vi "Without Data.vi"(8 "Error In":errorcluster, 11 "Communication In":refnum<class "Communication.lvclass">) -> (0 "Error Out":errorcluster, 3 "Communication Out":refnum<class "Communication.lvclass">)   [LabVIEW 2022 SP3, in "Communication.lvclass"]
doc: "This VI is an overriding method which notify the receiver without any data."
uses:
  Communication.lvclass
  Downloads/Sample PC Template/Sample PC Template/Typedefs/Data.ctl
  Downloads/Sample PC Template/Sample PC Template/Sample PC Template.lvlib
  Controls/User Event Operation.ctl
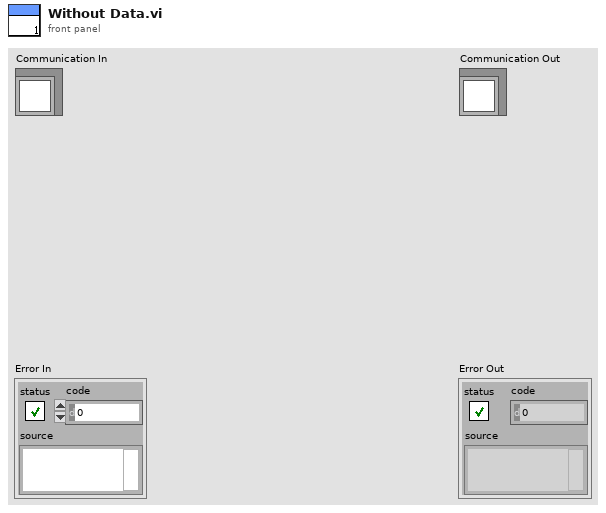
[diagram p1: front panel]
types:
  T1 = typedef "User Event Operation.ctl" = enum16{"Obtain", "Generate", "Release"}
  T2 = typedef "Sample PC Template.lvlib/Data.ctl" = cluster{"State":string, "Data":variant}
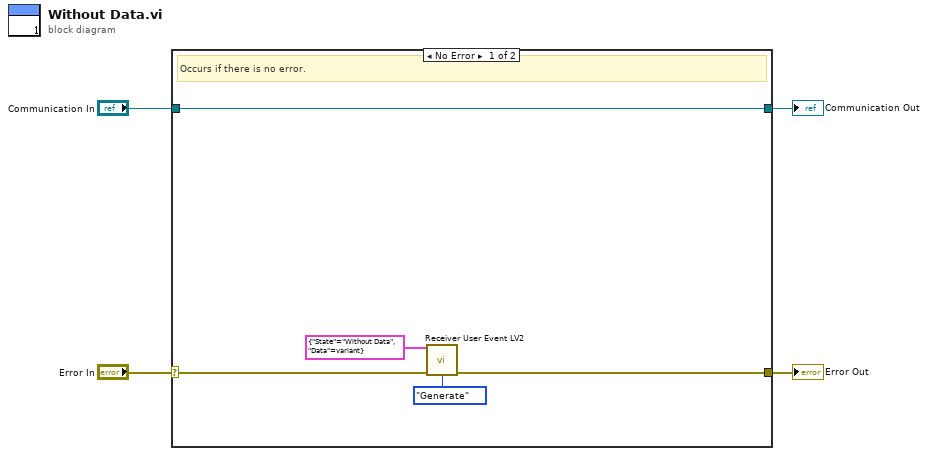
[diagram p0: block diagram]
diagram:
  n1 = case shown="No Error" "Error In" {
    selector: "Error In" -> [w8 w11]
    tunnel: [w7 w11] -> w3
    tunnel: [w9 w10] -> w1
    tunnel: "Communication In" -> [w9 w10]
    frame No Error {
      # "Occurs if there is no error."
      n2 = call "Receiver User Event LV2.vi"("Data"=T2 {"State"="Without Data", "Data"=variant}, "Error In"=w8, "Operation"=User_Event_Operation."Generate") -> ("Error Out"=w7:errorcluster)  [unwired: 11 in, 1 out]
    }
    frame Error {
      # "Occurs if there is any error."
    }
  }
  "Error Out" <- w3
  "Communication Out" <- w1
